vi "xml head.vi"(10 "TestResult":string, 11 "input_array_time":string[](array[string])) -> (3 "midVar_Content":string)   [LabVIEW 2011]
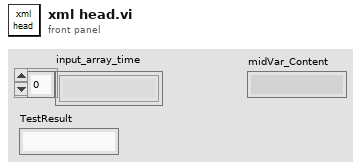
[diagram p1: front panel]
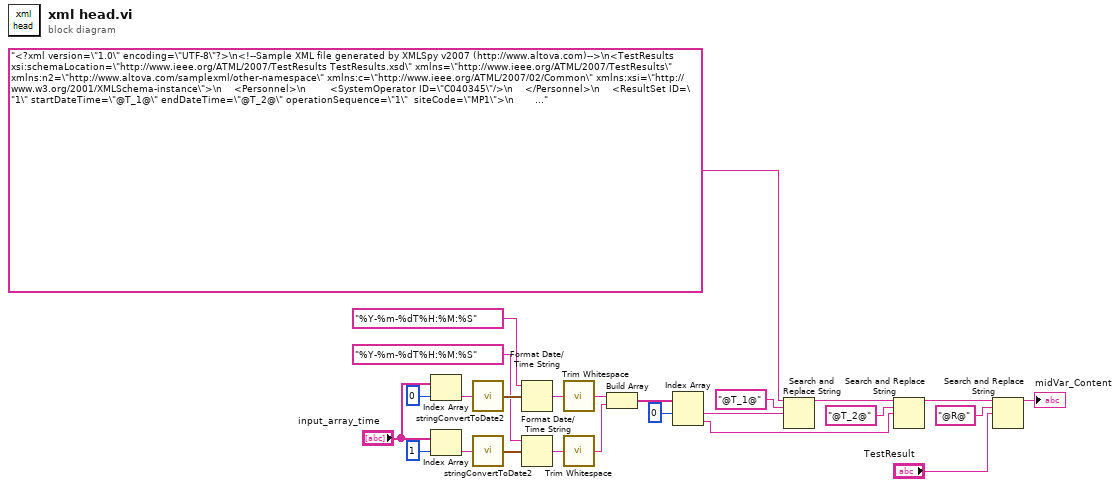
[diagram p0: block diagram]
diagram:
  n1 = Index Array(array="input_array_time", index=0 ("索引")) -> (element=w14:string)
  n2 = Index Array(array="input_array_time", index=1 ("索引")) -> (element=w13:string)
  n3 = call "stringConvertToDate2.vi"("input_str_yymmdd"=w14) -> ("show_date"=w11:timestamp)
  n4 = call "stringConvertToDate2.vi"("input_str_yymmdd"=w13) -> ("show_date"=w10:timestamp)
  n5 = Format Date/Time String(time format string (%c)="%Y-%m-%dT%H:%M:%S" ("时间格式字符串(%c)"), seconds (now)=w11) -> (date/time string=w17:string)  [unwired: 1 in]
  n6 = Format Date/Time String(time format string (%c)="%Y-%m-%dT%H:%M:%S" ("时间格式字符串(%c)"), seconds (now)=w10) -> (date/time string=w12:string)  [unwired: 1 in]
  n7 = call <vilib>:"Trim Whitespace.vi"("string"=w17) -> ("trimmed string"=w8:string)  [unwired: 1 in]
  n8 = call <vilib>:"Trim Whitespace.vi"("string"=w12) -> ("trimmed string"=w7:string)  [unwired: 1 in]
  n9 = Build Array(w8, w7) -> (w6:string[])
  n10 = Index Array(array=w6, index #1=0 ("索引")) -> (element #1=w23:string, element #2=w20:string)  [unwired: 1 in]
  n11 = Search and Replace String(input string="<?xml version=\"1.0\" encoding=\"UTF-8\"?>\n<!--Sample XML file generated by XMLSpy v2007 (http://www.altova.com)-->\n<TestResults xsi:schemaLocation=\"http://www.ieee.org/ATML/2007/TestResults TestResults.xsd\" xmlns=\"http://www.ieee.org/ATML/2007/TestResults\" xmlns:n2=\"http://www.altova.com/samplexml/other-namespace\" xmlns:c=\"http://www.ieee.org/ATML/2007/02/Common\" xmlns:xsi=\"http://www.w3.org/2001/XMLSchema-instance\">\n    <Personnel>\n        <SystemOperator ID=\"C040345\"/>\n    </Personnel>\n    <ResultSet ID=\"1\" startDateTime=\"@T_1@\" endDateTime=\"@T_2@\" operationSequence=\"1\"  siteCode=\"MP1\">\n        <Description>CMZ00A2R</Description>\n        <TestResult BoardFlag=\"1\" ID=\"1\">\n            <Outcome value=\"@R@\"/>\n        </TestResult>\n", search string="@T_1@" ("搜索字符串"), replace string=w23) -> (result string=w22:string)  [unwired: 5 in, 3 out]
  n12 = Search and Replace String(input string=w22, search string="@T_2@" ("搜索字符串"), replace string=w20) -> (result string=w5:string)  [unwired: 5 in, 3 out]
  n13 = Search and Replace String(input string=w5, search string="@R@" ("搜索字符串"), replace string="TestResult") -> (result string=→"midVar_Content":string)  [unwired: 5 in, 3 out]
